vi "FTW-TransferClient-dotNET-Callback-StatusDownload.vi"(4 "Initial Parameters":T1, 5 "Event Data":cluster{"sender":refnum<k24>, "e":refnum<k24>}, 6 "Control Ref":refnum<k24>, 7 "Event Common Data":T2) -> ()   [LabVIEW 2014, in "FTW-TransferClient-dotNET.lvclass"]
uses:
  FTW-TransferClient-dotNET.lvclass
  FTW-TransferClient-TransferStatus.ctl
  FTW-TransferClient.lvclass
panel:
  # "Inputs"
  # "Outputs"
  # "No Outputs - this VI\nis fire and forget"
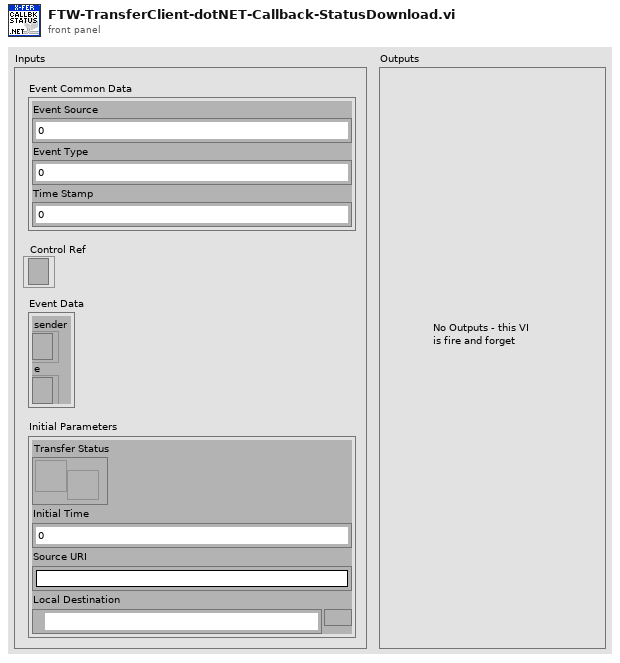
[diagram p1: front panel]
types:
  T1 = cluster{"Transfer Status":refnum<user-event>, "Initial Time":u32, "Source URI":string, "Local Destination":path}
  T2 = cluster{"Event Source":i32, "Event Type":u32, "Time Stamp":u32}
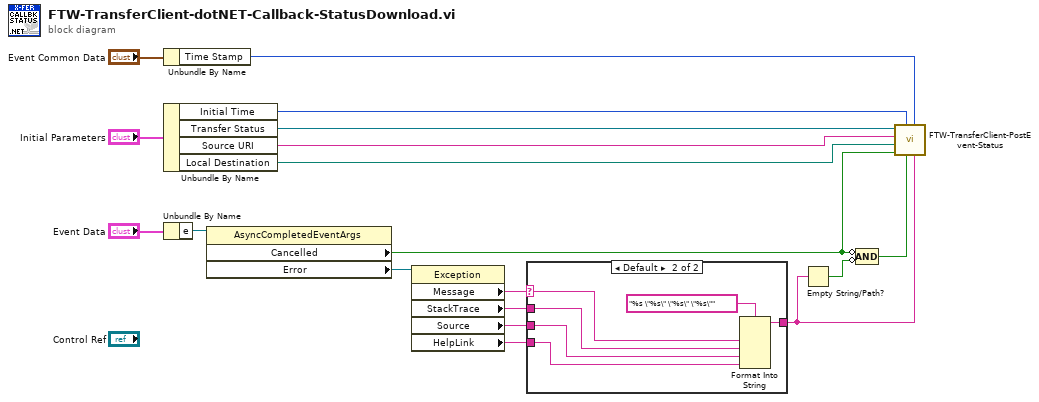
[diagram p0: block diagram]
diagram:
  n1 = Unbundle By Name("Event Common Data") -> ("Time Stamp"=w12:u32)
  n2 = Unbundle By Name("Initial Parameters") -> ("Initial Time"=w13:u32, "Transfer Status"=w14:refnum<user-event>, "Source URI"=w11:string, "Local Destination"=w10:path)
  n3 = Unbundle By Name("Event Data") -> ("e"=w15:refnum<k24>)
  n4 = property class="AsyncCompletedEventArgs"(reference=w15) -> ("Cancelled"=w9:bool, "Error"=w6:refnum<k24>)  [unwired: 1 in, 2 out]
  n5 = property class="Exception"(reference=w6) -> ("Message"=w4:string, "StackTrace"=w5:string, "Source"=w3:string, "HelpLink"=w2:string)  [unwired: 1 in, 2 out]
  n6 = case shown="Default" w4 {
    selector: w4 -> [_ w22]
    tunnel: w5 -> [_ w21]
    tunnel: [_ w23] -> w1
    tunnel: w3 -> [_ w20]
    tunnel: w2 -> [_ w19]
    frame "" {
    }
    frame Default {
      n7 = Format Into String(format string="%s \"%s\" \"%s\" \"%s\"", w22, w21, w20, w19) -> (resulting string=w23:string)  [unwired: 2 in, 1 out]
    }
  }
  n8 = Empty String/Path?(string/path=w1) -> (empty?=w8:bool)
  n9 = Compound Arithmetic op=AND(invert w9, invert w8) -> (w7:bool)
  n10 = call "FTW-TransferClient-PostEvent-Status.vi"("Error Message"=w1, "Timestamp"=w12, "Error?"=w7, "Initial Timestamp"=w13, "Cancelled?"=w9, "Local Filepath"=w10, "Remote URI"=w11, "Transfer Status Event"=w14) -> ()  [unwired: 4 in]
